vi "clusterTypesExample.vi"() -> ()   [LabVIEW 2014]
panel:
  out "Modfied Cluster Indicator":T1
  out "Cluster Indicator":T1
  in  "Simple 4-Vector":cluster{"X":dbl, "Y":dbl, "Z":dbl, "T":dbl}
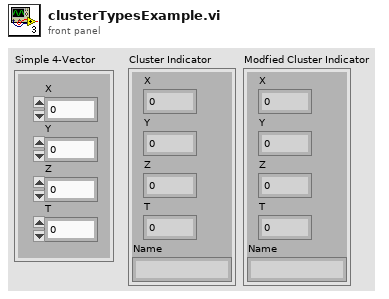
[diagram p1: front panel]
types:
  T1 = cluster{"X":dbl, "Y":dbl, "Z":dbl, "T":dbl, "Name":string}
  T2 = cluster{"X":dbl, "T":dbl, "Y":dbl, "Z":dbl, "Name":string}
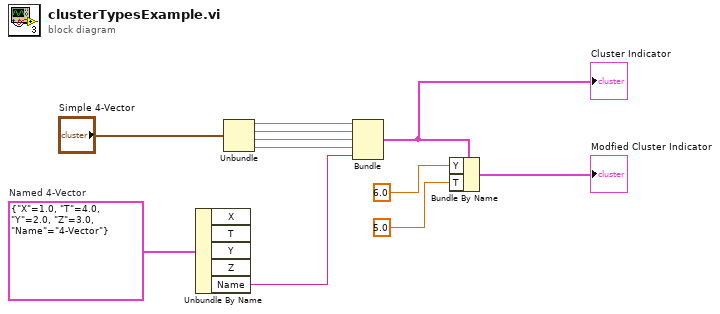
[diagram p0: block diagram]
diagram:
  w11 = T2 {"X"=1.0, "T"=4.0, "Y"=2.0, "Z"=3.0, "Name"="4-Vector"}  # Named 4-Vector
  n1 = Unbundle By Name "Unbundle By Name"(w11) -> ("Name"=w5:string)  [unwired: 4 out]
  n2 = Unbundle "Unbundle"("Simple 4-Vector") -> ("X"=w9:dbl, "Y"=w8:dbl, "Z"=w7:dbl, "T"=w6:dbl)
  n3 = Bundle "Bundle"("X"=w9, "Y"=w8, "Z"=w7, "T"=w6, "Name"=w5) -> (w4:T1)  [unwired: 1 in]
  "Cluster Indicator" <- w4
  n4 = Bundle By Name "Bundle By Name"(cluster=w4, "Y"=6.0, "T"=5.0) -> (→"Modfied Cluster Indicator":T1)
